vi "Read data file (SubVI).vi"(7 "format (%.;%.7e)":string="%.;%.7e", 8 "error in":errorcluster, 9 "Binary":bool, 11 "file path in":path) -> (0 "error out":errorcluster, 1 "Number of columns":i32, 2 "2D data":dbl[][](array[numeric]), 3 "file path out":path)   [LabVIEW 2019]
doc: "Reads data from a data file (binary or text based)"
uses:
  <vilib>/Utility/file.llb/Read Delimited Spreadsheet (DBL).vi
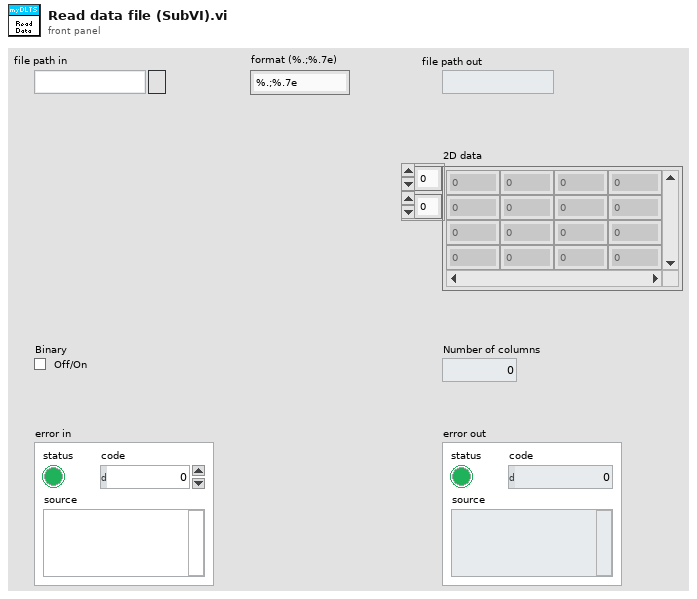
[diagram p1: front panel]
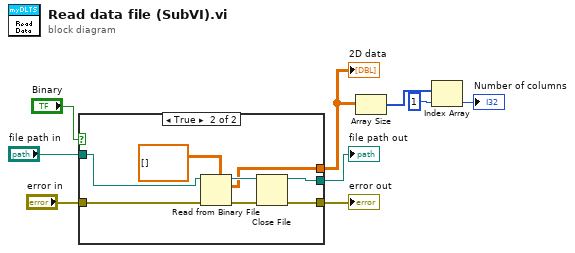
[diagram p0: block diagram]
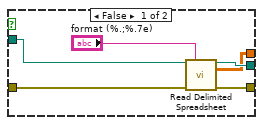
[diagram p2: hidden frame]
diagram:
  n1 = case shown="True" "Binary" {
    tunnel: "file path in" -> [w14 w23]
    tunnel: "error in" -> [w15 w22]
    tunnel: [w11 w19] -> w5
    tunnel: [w12 w18] -> w6
    tunnel: [w10 w16] -> w4
    frame False {
      n2 = call-poly <vilib>:"Read Delimited Spreadsheet.vi"("file path (dialog if empty)"=w14, "format (%.3f)"="format (%.;%.7e)", "error in (no error)"=w15) -> ("new file path (Not A Path if cancelled)"=w12:path, "all rows"=w10:dbl[][], "error out"=w11:errorcluster)  [unwired: 7 in, 3 out]
    }
    frame True {
      n3 = Read from Binary File(5:dbl[][] [] ("2D data"), 8:w22, 11:w23) -> (0:w20:errorcluster, 2:w16:dbl[][], 3:w21:refnum<file>)  [unwired: 3 in, 1 out]
      n4 = Close File(refnum=w21, error in=w20) -> (path=w18:path, error out=w19:errorcluster)
    }
  }
  "file path out" <- w6
  "error out" <- w5
  "2D data" <- w4
  n5 = Array Size(array=w4) -> (size(s)=w3:i32[])
  n6 = Index Array(array=w3, index=1) -> (element=→"Number of columns":i32)
